vi "Perform Work.vi"(8 "error in (no error)":errorcluster, 9 "Initialize":bool, 10 "Reply to":refnum<class "Result Reply Msg.lvclass">, 11 "Measure Object in":refnum<class "Worker.lvclass">) -> (0 "error out":errorcluster, 3 "Measure Object out":refnum<class "Worker.lvclass">)   [LabVIEW 2016, in "Worker.lvclass"]
uses:
  Worker.lvclass
  D:/github/Measure_core/Da Base/Da Base.lvclass
  Da Base Messages/Result Reply Msg/Result Reply Msg.lvclass
  Da Base/Da Base.lvclass/Da Base.ctl
  Worker.lvclass/Worker.ctl
  da Base/Write Reply to.vi
  da Base/Write Active.vi
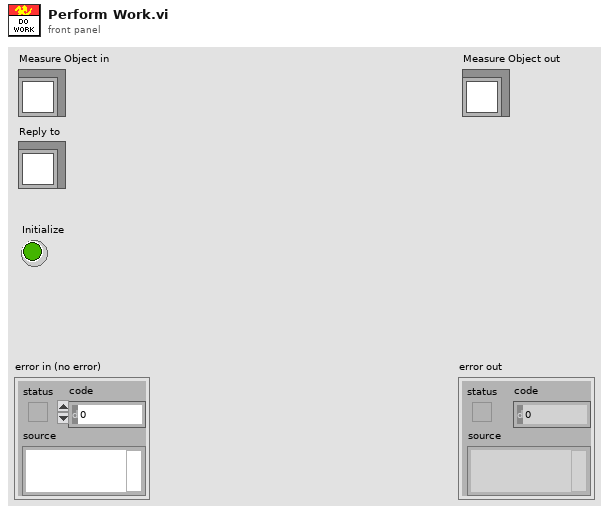
[diagram p1: front panel]
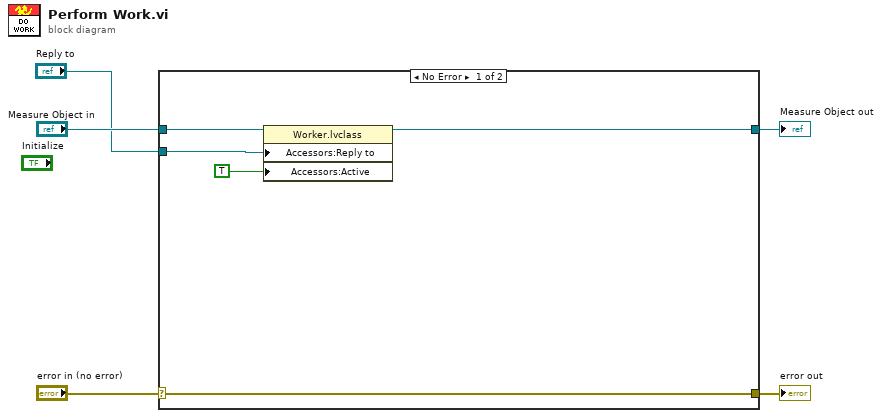
[diagram p0: block diagram]
diagram:
  n1 = case shown="No Error" "error in (no error)" {
    selector: "error in (no error)" -> [w9 w12]
    tunnel: [w9 w12] -> w4
    tunnel: [w8 w11] -> w2
    tunnel: "Measure Object in" -> [w10 w11]
    tunnel: "Reply to" -> [w7 _]
    frame No Error {
      n2 = property class="Worker.lvclass"(reference=w10, "Accessors:Reply to"=w7, "Accessors:Active"=TRUE ("Active")) -> (reference out=w8:refnum<class "Worker.lvclass">)  [unwired: 1 in, 1 out]
    }
    frame Error {
    }
  }
  "error out" <- w4
  "Measure Object out" <- w2
